vi "Multi-Button Toggle.vi"(8 "Button 4":bool, 9 "Button 3":bool, 10 "Button 2":bool, 11 "Button 1":bool) -> (3 "Output":bool)   [LabVIEW 2017]
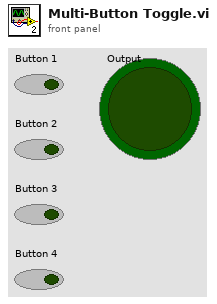
[diagram p1: front panel]
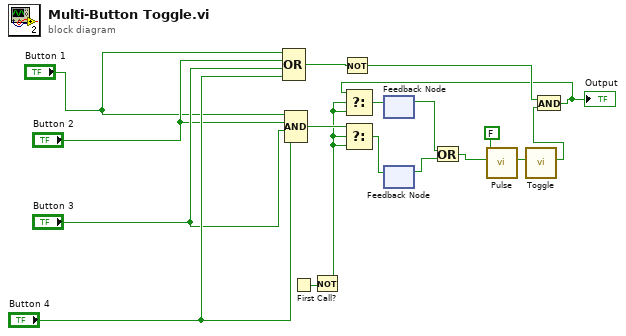
[diagram p0: block diagram]
diagram:
  n1 = Compound Arithmetic op=OR("Button 1", "Button 2", "Button 3", "Button 4") -> (w13:bool)
  n2 = Compound Arithmetic op=AND("Button 1", "Button 2", "Button 3", "Button 4") -> (w6:bool)
  n3 = First Call?() -> (First Call?: T/F=w2:bool)
  n4 = Not(x=w2) -> (.not. x?=w1:bool)
  n5 = Not(x=w13) -> (.not. x?=w15:bool)
  n6 = Select(t=w6, s=w1, f=w1) -> (s? t:f=w5:bool)
  n7 = feedback #1() -> (w17:bool)  [unwired: 1 in]
  n8 = feedback #2() -> (w16:bool)  [unwired: 1 in]
  n9 = feedback-in #2(w5) -> ()
  n10 = Or(x=w17, y=w16) -> (x .or. y?=w18:bool)
  n11 = call "Pulse.vi"("Input"=w18, "Rising Edge?"=FALSE) -> ("Output"=w7:bool)  [unwired: 9 in]
  n12 = call "Toggle.vi"("Input"=w7) -> ("Output"=w14:bool)  [unwired: 10 in]
  n13 = And(x=w15, y=w14) -> (x .and. y?=w4:bool)
  "Output" <- w4
  n14 = Select(t=w4, s=w1, f=w1) -> (s? t:f=w3:bool)
  n15 = feedback-in #1(w3) -> ()
